vi "Set Reentrant.vi"(8 "error in (no error)":errorcluster, 10 "reentrant":bool, 11 "measurement in":refnum<class "Continuous Counting Measurement.lvclass">) -> (0 "error out":errorcluster, 3 "measurement out":refnum<class "Continuous Counting Measurement.lvclass">)   [LabVIEW 2021, in "MeasurementServerTests.lvlib" / "Measurement Service Tests.lvlib" / "Continuous Counting Measurement.lvclass"]
uses:
  Continuous Counting Measurement.lvclass
  Continuous Counting Measurement.lvclass/Continuous Counting Measurement.ctl
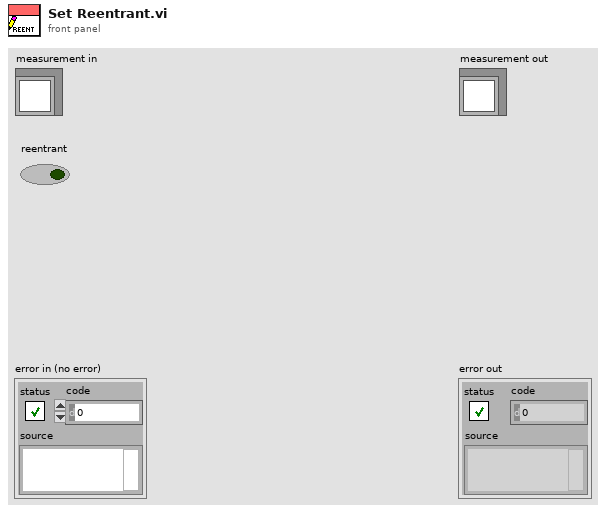
[diagram p1: front panel]
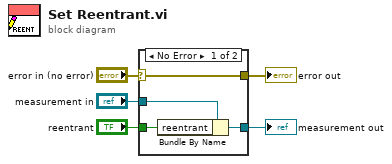
[diagram p0: block diagram]
diagram:
  n1 = case shown="No Error" "error in (no error)" {
    selector: "error in (no error)" -> [w9 w10]
    tunnel: [w9 w10] -> w4
    tunnel: [w7 w11] -> w2
    tunnel: "measurement in" -> [w8 w11]
    tunnel: "reentrant" -> [w6 _]
    frame No Error {
      n2 = Bundle By Name(cluster=w8, "reentrant"=w6) -> (w7:refnum<class "Continuous Counting Measurement.lvclass">)
    }
    frame Error {
    }
  }
  "error out" <- w4
  "measurement out" <- w2
